vi "SaveTimestampedFPpng.vi"(9 "seconds since 1Jan1904":timestamp format="%<%Y-%m-%d-%H-%M-%S>T", 10 "FolderName":string, 11 "VIpath":path) -> (3 "File Path Out":path)   [LabVIEW 2022 SP3]
panel:
  out "error out":errorcluster
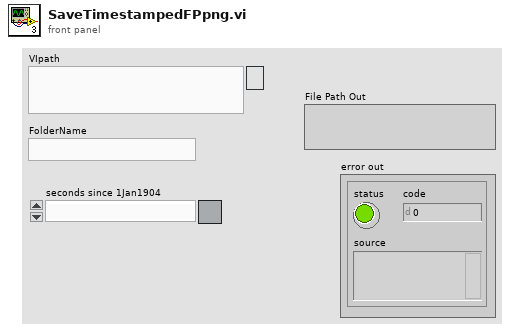
[diagram p1: front panel]
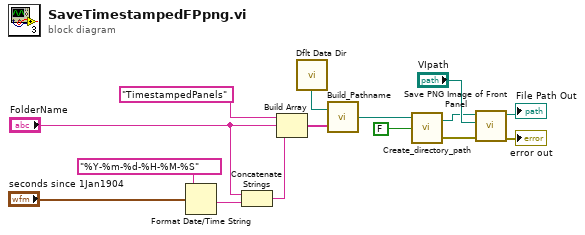
[diagram p0: block diagram]
diagram:
  n1 = Format Date/Time String(time format string (%c)="%Y-%m-%d-%H-%M-%S", seconds (now)="seconds since 1Jan1904") -> (date/time string=w15:string)  [unwired: 1 in]
  n2 = Concatenate Strings("FolderName", w15) -> (w4:string)
  n3 = Build Array("TimestampedPanels" ("element"), "FolderName", w4) -> (w6:string[])
  n4 = call <vilib>:"Dflt Data Dir.vi"() -> ("App:Default Data Directory"=w7:path)
  n5 = call "Build_Pathname.vi"("PathElements"=w6, "PathnameIn"=w7) -> ("AppendedPath"=w3:path)
  n6 = call "Create_directory_path.vi"("Dialog Box"=FALSE, "Path name"=w3) -> ("error out"=w8:errorcluster, "Path name Out"=w1:path)  [unwired: 1 in]
  n7 = call "Save PNG Image of Front Panel.vi"("error in (no error)"=w8, "VI Path"="VIpath", "File Path In"=w1) -> ("error out"=→"error out":errorcluster, "File Path Out"=→"File Path Out":path)  [unwired: 7 in]
